vi "Panel Set GUI Builder Director.vi"(8 "error in (no error)":errorcluster, 10 "GUI Control Builder Director.lvclass":refnum<class "GUI Control Builder Director.lvclass">, 11 "Panel in":refnum<class "Panel Controller Interface.lvclass">) -> (0 "error out":errorcluster, 3 "Panel out":refnum<class "Panel Controller Interface.lvclass">)   [LabVIEW 2015, in "EditPanel API.lvlib" / "Panel Controller Interface.lvclass"]
uses:
  Panel Controller Interface.lvclass
  myPanel/GUI/GUI Builder Director/GUI Control Builder Director.lvclass
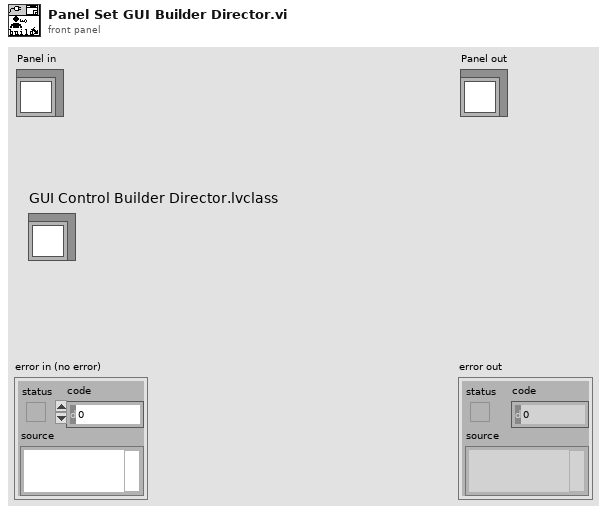
[diagram p1: front panel]
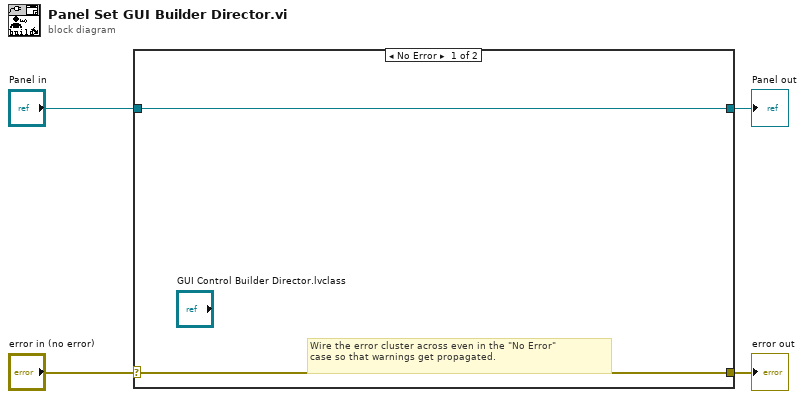
[diagram p0: block diagram]
diagram:
  n1 = case shown="No Error" "error in (no error)" {
    selector: "error in (no error)" -> [w5 w8]
    tunnel: [w5 w8] -> w3
    tunnel: [w6 w7] -> w1
    tunnel: "Panel in" -> [w6 w7]
    frame No Error {
      # "Wire the error cluster across even in the \"No Error\"\ncase so that warnings get propagated."
    }
    frame Error {
    }
  }
  "error out" <- w3
  "Panel out" <- w1
